vi "CheckCmdsDummy.vi"(0 "scanChanged":bool, 1 "actScan":i32, 2 "stepChanged":bool, 3 "actStep":i32, 5 "outbit_iN":bool, 9 "CMD array":u32[](array[numeric]) format="%032b") -> (19 "outbit_out":bool)   [LabVIEW 2014]
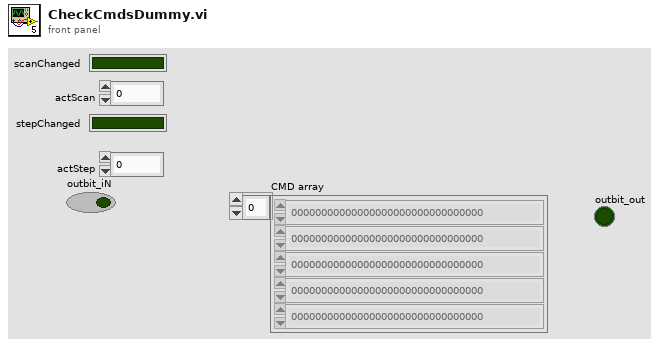
[diagram p1: front panel]
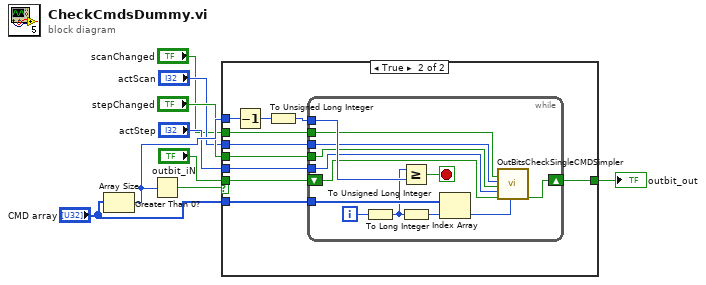
[diagram p0: block diagram]
diagram:
  n1 = Array Size(array="CMD array") -> (size(s)=w7:i32)
  n2 = Greater Than 0?(x=w7) -> (x > 0?=w8:bool)
  n3 = case shown="True" w8 {
    tunnel: "CMD array" -> [_ w20]
    tunnel: w7 -> [_ w19]
    tunnel: "outbit_iN" -> [w10 w16]
    tunnel: [w10 w11] -> w6
    tunnel: "actStep" -> [_ w15]
    tunnel: "stepChanged" -> [_ w14]
    tunnel: "actScan" -> [_ w13]
    tunnel: "scanChanged" -> [_ w12]
    frame False {
    }
    frame True {
      n4 = Decrement(x=w19) -> (x-1=w17:i32)
      n5 = To Unsigned Long Integer(number=w17) -> (unsigned 32bit integer=w18:u32)
      n6 = while {
        tunnel: w18 -> [w32]
        tunnel: w20 -> [w30]
        tunnel: w15 -> [w25]
        tunnel: w14 -> [w24]
        tunnel: w13 -> [w23]
        tunnel: w12 -> [w22]
        shift-right: [w21] -> w11
        shift-left: w16 -> [w29]
        i -> [w33]
        stop <- w31 stop-if-true
        n7 = To Unsigned Long Integer(number=w33) -> (unsigned 32bit integer=w27:u32)
        n8 = Greater Or Equal?(x=w27, y=w32) -> (x >= y?=w31:bool)
        n9 = To Long Integer(number=w27) -> (32bit integer=w26:i32)
        n10 = Index Array(array=w30, index=w26) -> (element=w28:u32)
        n11 = call "OutBitsCheckSingleCMDSimpler.vi"("scanChanged"=w22, "actScan"=w23, "stepChanged"=w24, "actStep"=w25, "outbit_in"=w29, "CMDin"=w28) -> ("outbit_out"=w21:bool)  [unwired: 13 in]
      }
    }
  }
  "outbit_out" <- w6
